vi "Get Transfer Buffers.vi"(8 "error in (no error)":errorcluster, 11 "Transfer in":refnum<class "Transfer.lvclass">) -> (0 "error out":errorcluster, 1 "string Buffer":refnum<class "Buffer.lvclass">, 2 "engine Buffer":refnum<class "Buffer.lvclass">, 3 "Transfer out":refnum<class "Transfer.lvclass">)   [LabVIEW 2021, in "DSF Core.lvlib" / "Transfer.lvclass"]
uses:
  Transfer.lvclass
  Buffer/Buffer.lvclass
  Transfer.lvclass/Transfer.ctl
  Buffers/Buffers.lvclass/Buffers.ctl
  Buffers/Buffers.lvclass
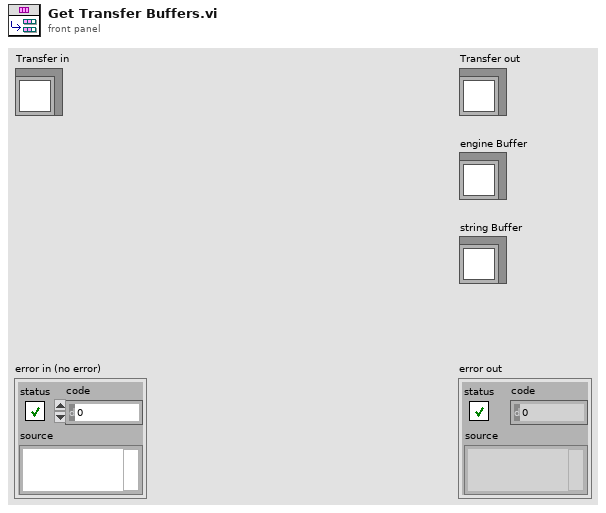
[diagram p1: front panel]
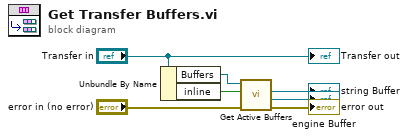
[diagram p0: block diagram]
diagram:
  n1 = Unbundle By Name("Transfer in") -> ("Buffers"=w6:refnum<class "Buffers.lvclass">, "inline"=w3:bool)
  n2 = call "Get Active Buffers.vi"("error in (no error)"="error in (no error)", "inline?"=w3, "Buffers in"=w6) -> ("error out"=→"error out":errorcluster, "engine Buffer"=→"engine Buffer":refnum<class "Buffer.lvclass">, "string Buffer"=→"string Buffer":refnum<class "Buffer.lvclass">)  [unwired: 5 in, 1 out]
  "Transfer out" <- "Transfer in"
